vi "Value to String.vi"(8 "error in (no error)":errorcluster, 11 "NT Scalar in":refnum<class "NT Scalar.lvclass">) -> (0 "error out":errorcluster, 2 "string":string, 3 "NT Scalar out":refnum<class "NT Scalar.lvclass">)   [LabVIEW 2020, in "PV Access.lvlib" / "PV Data.lvlib" / "NT Scalar.lvclass"]
uses:
  NT Scalar.lvclass
  NT Scalar.lvclass/NT Scalar.ctl
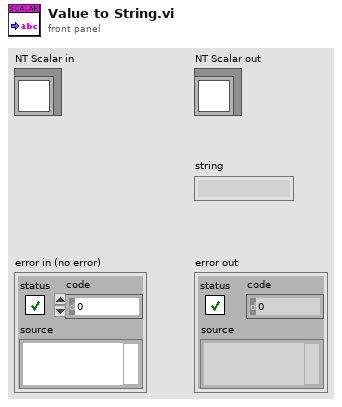
[diagram p1: front panel]
types:
  T1 = typedef "PV Access.lvlib/PV Data.lvlib/Type Code.ctl" = enum8{"Null", "Bool", "BoolA", "Int8", "Int8A", "Int16", "Int16A", "Int32", "Int32A", "Int64", "Int64A", "UInt8", "UInt8A", "UInt16", "UInt16A", "UInt32", "UInt32A", "UInt64", "UInt64A", "Float32", "Float32A", "Float64", "Float64A", "String", "StringA", "Struct", "StructA", "Union", "UnionA", "Any", "AnyA"}
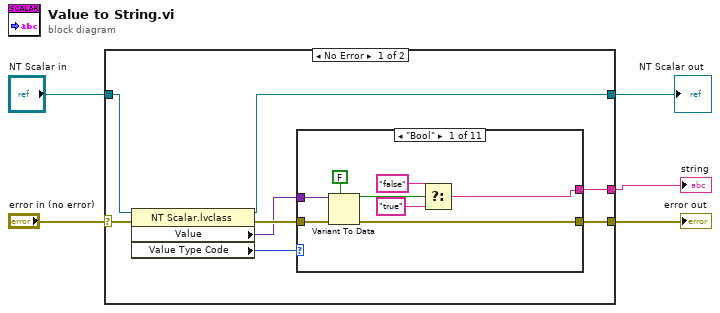
[diagram p0: block diagram]
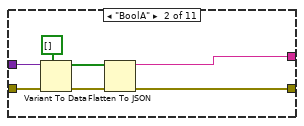
[diagram p2: hidden frame]
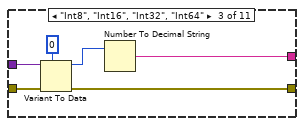
[diagram p3: hidden frame]
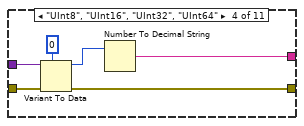
[diagram p4: hidden frame]
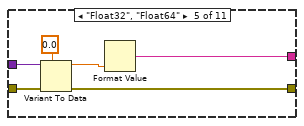
[diagram p5: hidden frame]
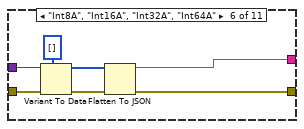
[diagram p6: hidden frame]
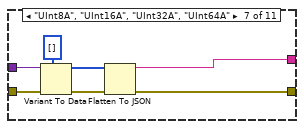
[diagram p7: hidden frame]
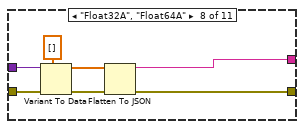
[diagram p8: hidden frame]
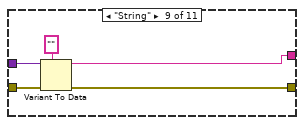
[diagram p9: hidden frame]
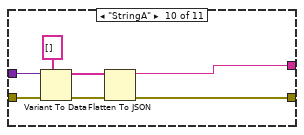
[diagram p10: hidden frame]
diagram:
  n1 = case shown="No Error" "error in (no error)" {
    selector: "error in (no error)" -> [w7 w82]
    tunnel: [w6 w82] -> w3
    tunnel: [w11 w81] -> w1
    tunnel: "NT Scalar in" -> [w13 w81]
    tunnel: [w8 _] -> w2
    frame No Error {
      n2 = property class="NT Scalar.lvclass"(reference=w13, error in=w7) -> (reference out=w11:refnum<class "NT Scalar.lvclass">, error out=w12:errorcluster, "Value"=w9:variant, "Value Type Code"=w10:T1)
      n3 = case shown="\"Bool\"" w10 {
        tunnel: w12 -> [w20 w27 w32 w38 w44 w52 w59 w66 w71 w78 w80]
        tunnel: w9 -> [w21 w28 w33 w39 w45 w53 w60 w67 w72 w79 _]
        tunnel: [w19 w23 w29 w35 w42 w48 w54 w62 w70 w74 w80] -> w6
        tunnel: [w14 w22 w31 w37 w43 w47 w55 w61 w68 w73 _] -> w8
        frame "Bool" {
          n4 = Variant To Data(error in=w20, type=FALSE, Variant=w21) -> (data=w17:bool, error out=w19:errorcluster)
          n5 = Select(t="false", s=w17, f="true") -> (s? t:f=w14:string)
        }
        frame "BoolA" {
          n6 = Variant To Data(error in=w27, type=bool[] [], Variant=w28) -> (data=w24:bool[], error out=w25:errorcluster)
          n7 = Flatten To JSON(anything=w24, error in (no error)=w25) -> (JSON string=w22:string, 11:w23:errorcluster)  [unwired: 1 in]
        }
        frame "Int8", "Int16", "Int32", "Int64" {
          n8 = Variant To Data(error in=w32, type=i64 0, Variant=w33) -> (data=w30:i64, error out=w29:errorcluster)
          n9 = Number To Decimal String(number=w30) -> (decimal integer string=w31:string)  [unwired: 1 in]
        }
        frame "UInt8", "UInt16", "UInt32", "UInt64" {
          n10 = Variant To Data(error in=w38, type=u64 0, Variant=w39) -> (data=w36:u64, error out=w35:errorcluster)
          n11 = Number To Decimal String(number=w36) -> (decimal integer string=w37:string)  [unwired: 1 in]
        }
        frame "Float32", "Float64" {
          n12 = Variant To Data(error in=w44, type=0.0, Variant=w45) -> (data=w41:dbl, error out=w42:errorcluster)
          n13 = Format Value(value (0)=w41) -> (output string=w43:string)  [unwired: 2 in]
        }
        frame "Int8A", "Int16A", "Int32A", "Int64A" {
          n14 = Variant To Data(error in=w52, type=i64[] [], Variant=w53) -> (data=w49:i64[], error out=w50:errorcluster)
          n15 = Flatten To JSON(anything=w49, error in (no error)=w50) -> (JSON string=w47:string, 11:w48:errorcluster)  [unwired: 1 in]
        }
        frame "UInt8A", "UInt16A", "UInt32A", "UInt64A" {
          n16 = Variant To Data(error in=w59, type=u64[] [], Variant=w60) -> (data=w56:u64[], error out=w57:errorcluster)
          n17 = Flatten To JSON(anything=w56, error in (no error)=w57) -> (JSON string=w55:string, 11:w54:errorcluster)  [unwired: 1 in]
        }
        frame "Float32A", "Float64A" {
          n18 = Variant To Data(error in=w66, type=dbl[] [], Variant=w67) -> (data=w63:dbl[], error out=w64:errorcluster)
          n19 = Flatten To JSON(anything=w63, error in (no error)=w64) -> (JSON string=w61:string, 11:w62:errorcluster)  [unwired: 1 in]
        }
        frame "String" {
          n20 = Variant To Data(error in=w71, type="", Variant=w72) -> (data=w68:string, error out=w70:errorcluster)
        }
        frame "StringA" {
          n21 = Variant To Data(error in=w78, type=string[] [], Variant=w79) -> (data=w75:string[], error out=w76:errorcluster)
          n22 = Flatten To JSON(anything=w75, error in (no error)=w76) -> (JSON string=w73:string, 11:w74:errorcluster)  [unwired: 1 in]
        }
        frame Default {
        }
      }
    }
    frame Error {
    }
  }
  "error out" <- w3
  "NT Scalar out" <- w1
  "string" <- w2
